vi "Append_to_file.vi"(8 "error in":errorcluster, 9 "file path (use dialog)":path=path "C:/Users/Guest_2/Desktop/Zong Long/Data trial.txt", 10 "text":string) -> (0 "error out":errorcluster)   [LabVIEW 2015]
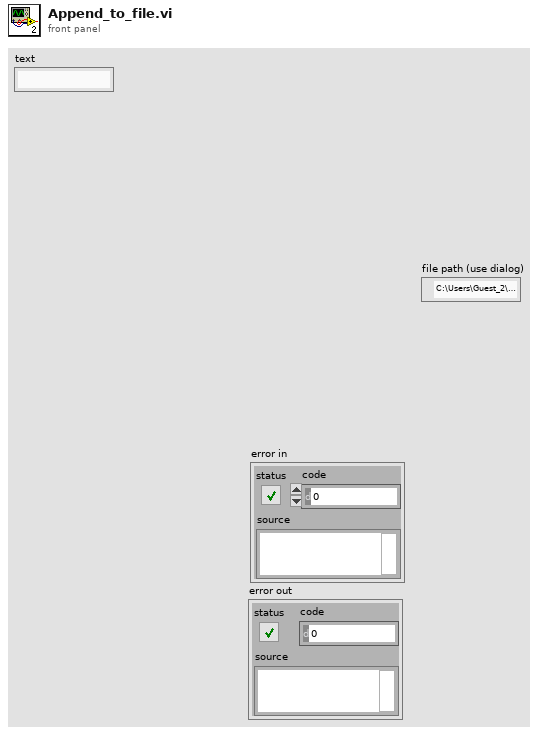
[diagram p1: front panel]
types:
  T1 = enum16{"open", "replace", "create", "open or create", "replace or create", "replace or create with confirmation"}
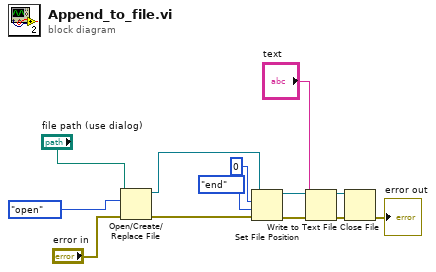
[diagram p0: block diagram]
diagram:
  n1 = Open/Create/Replace File(file path (use dialog)="file path (use dialog)", error in="error in", operation (0:open)=T1."open") -> (refnum out=w7:refnum<file>, error out=w9:errorcluster)  [unwired: 3 in, 1 out]
  n2 = Set File Position(offset (in bytes) (0)=i64 0, refnum=w7, from (0:start)=enum16{"start", "end", "current"}."end", error in=w9) -> (refnum out=w5:refnum<file>, error out=w6:errorcluster)
  n3 = Write to Text File(file (use dialog)=w5, text="text", error in=w6) -> (refnum out=w3:refnum<file>, error out=w4:errorcluster)  [unwired: 1 in, 1 out]
  n4 = Close File(refnum=w3, error in=w4) -> (error out=→"error out":errorcluster)  [unwired: 1 out]
